vi "DTB_4848_RTU.vi"() -> ()   [LabVIEW 2020]
uses:
  <vilib>/Instr/_visa.llb/VISA Configure Serial Port (Instr).vi
panel:
  in  "Select Device":u16(ring) items=["Broadcast", "DTB4848 1st", "DTB4848 2nd"]
  in  "Boolean 2":bool
  in  "Boolean 3":bool
  in  "Boolean 4":bool
  in  "Boolean 5":bool
  in  "Boolean 6":bool
  in  "Boolean 7":bool
  in  "Boolean 8":bool
  in  "Boolean 9":bool
  in  "Set Point":dbl
  in  "Mode Control":u16
  in  "Ti Integral time":dbl
  in  "Control Cycle 1st":dbl
  in  "Control Cycle 2nd":dbl
  in  "PB Proportional band":dbl
  in  "Td Derivative time":dbl
  in  "Proportional control\noffset error value":dbl
  out "Process Value":dbl
  out "Set Point":dbl
  out "PB Proportional band":dbl
  out "Proportional control\noffset error value":dbl
  out "Control method":u16=13
  out "Ti Integral time":u16=13
  out "Td Derivative time":u16=13
  out "Control Cycle 1st":dbl
  out "Control Cycle 2nd":dbl
  out "Process Value":dbl
  out "Set Point":dbl
  out "PB Proportional band":dbl
  out "Proportional control\noffset error value":dbl
  out "Control method":u16=13
  out "Ti Integral time":u16=13
  out "Td Derivative time":u16=13
  out "Control Cycle 1st":dbl
  out "Control Cycle 2nd":dbl
  out "k":i32
  out "x = 0?":bool
  in  "stop":bool
  in  "Cluster":T1={"VISA resource name"="COM1", "Baud rate"=9600, "Data bits"=8, "Parity"=enum."None", "Stop bits"=10, "Flow control"=0, "Timeout"=1000, "Termination char\n(0xA = '\\n' = LF) "=10, "Enable Termination\nChar (T)"=TRUE} {"Termination char\n(0xA = '\\n' = LF)" format="%.0x"; "Flow control" items=["None", "XON/XOFF", "RTS/CTS", "XON/XOFF & RTS/CTS", "DTR/DSR", "XON/XOFF & DTR/DSR"]; "Stop bits" items=["1.0"=10, "1.5"=15, "2.0"=20]; "Data bits" min=5 max=8 step=1}
  in  "Set":bool
  # "HE THONG DIEU KHIEN GIAM SAT THIET BI DIEU KHIEN NHIET DO DTB4848"
  # "CAU HINH\nTRUYEN THONG"
  # "THIET LAP\nGIA TRI THAM SO"
  # "DTB4848\nDEVICE 1"
  # "DTB4848\nDEVICE 2"
  # "HANH DONG"
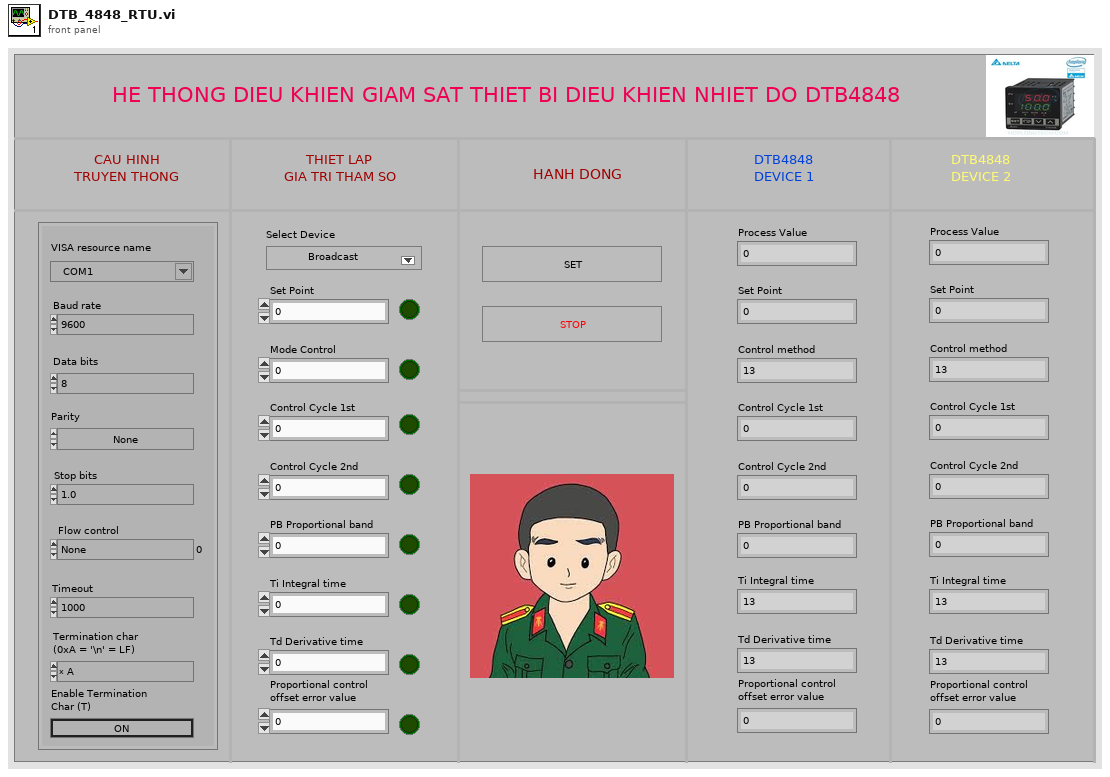
[diagram p1: front panel]
types:
  T1 = cluster{"VISA resource name":refnum<visa-resource-name>, "Baud rate":u32, "Data bits":u16, "Parity":enum16{"None", "Odd", "Even", "Mark", "Space"}, "Stop bits":u16, "Flow control":u16, "Timeout":u32, "Termination char\n(0xA = '\\n' = LF) ":u8, "Enable Termination\nChar (T)":bool}
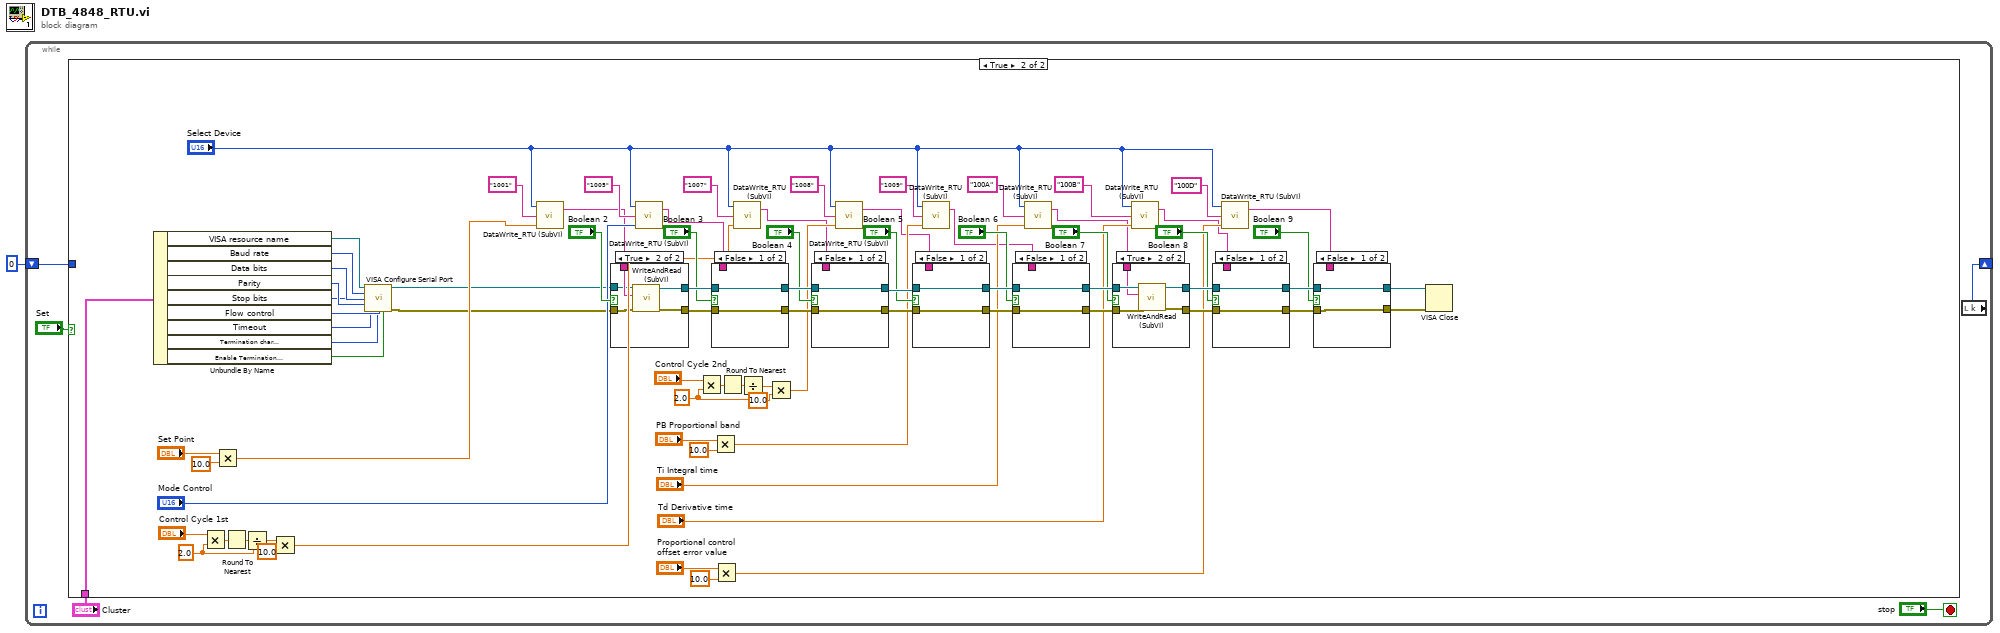
[diagram p0: block diagram]
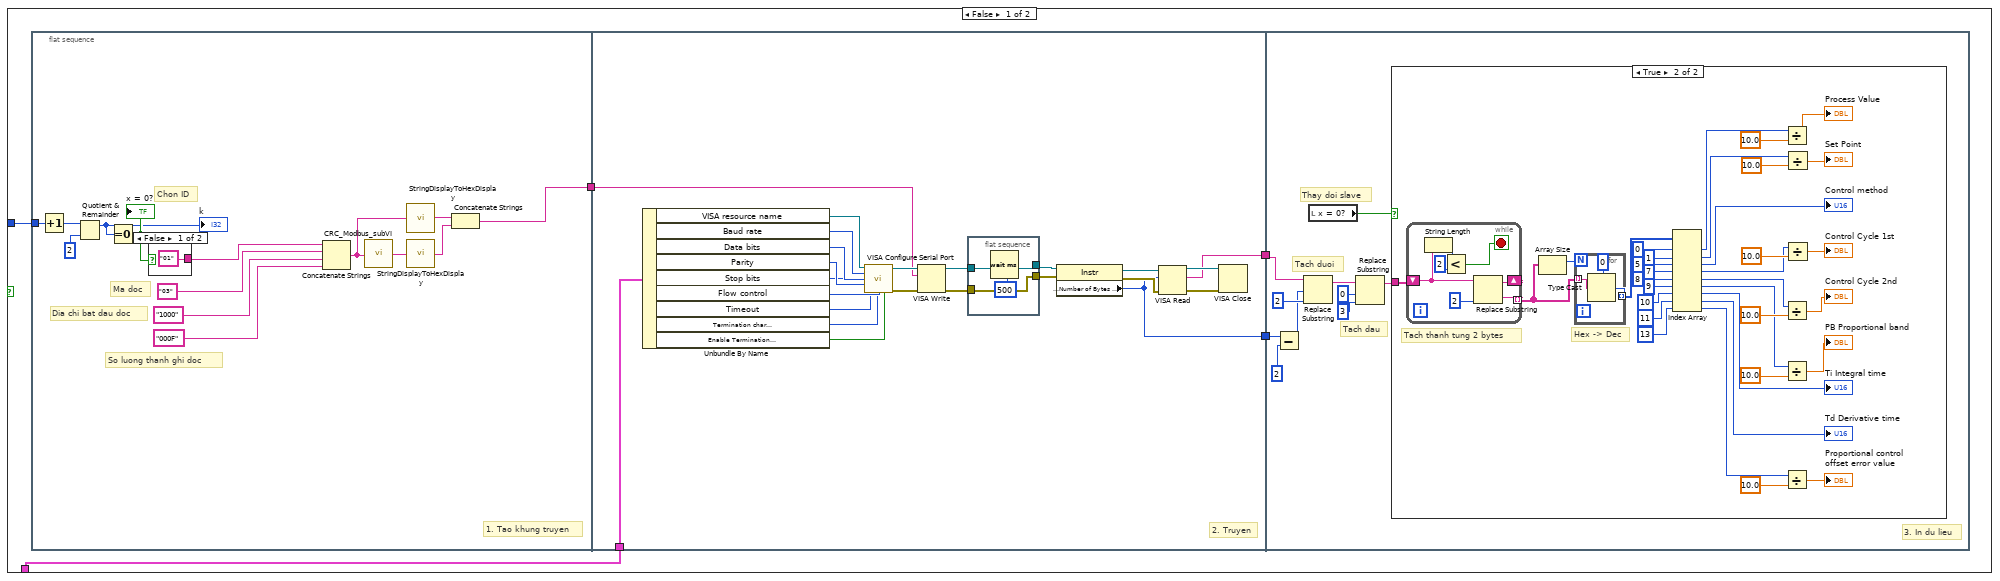
[diagram p2: hidden frame]
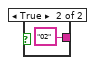
[diagram p3: hidden frame]
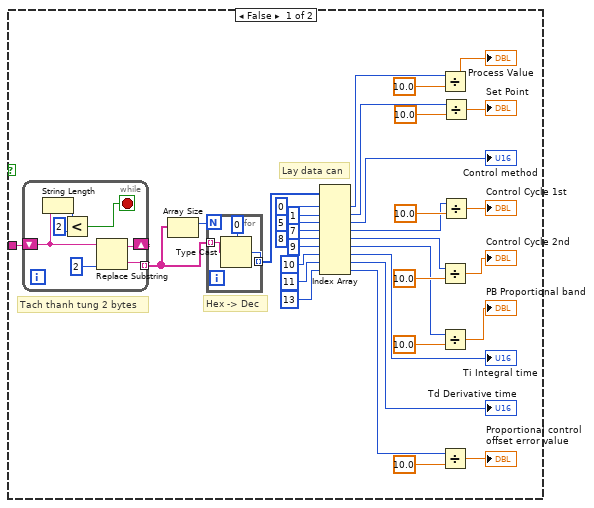
[diagram p4: hidden frame]
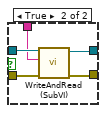
[diagram p5: hidden frame]
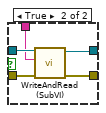
[diagram p6: hidden frame]
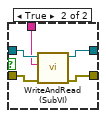
[diagram p8: hidden frame]
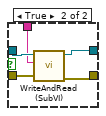
[diagram p9: hidden frame]
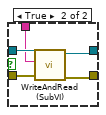
[diagram p10: hidden frame]
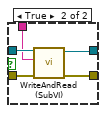
[diagram p11: hidden frame]
diagram:
  n1 = while {
    shift-right: [w5] -> _
    shift-left: 0 ("k") -> [w6]
    stop <- "stop" stop-if-true
    n2 = case shown="True" "Set" {
      tunnel: w6 -> [w11 _]
      tunnel: "Cluster" -> [w10 w230]
      frame False {
        n3 = flat-sequence {
          tunnel: w11 -> [w22]
          tunnel: [w12] -> w7
          tunnel: w10 -> [w31]
          tunnel: [w30] -> w9
          tunnel: [w29] -> w8
          tunnel: w7 -> [w28]
          tunnel: w9 -> [w62]
          tunnel: w8 -> [w56]
          frame #0 {
            # "1. Tao khung truyen"
            # "Chon ID"
            # "So luong thanh ghi doc"
            # "Dia chi bat dau doc"
            # "Ma doc"
            n4 = Increment(x=w22) -> (x+1=w21:i32)
            n5 = Quotient & Remainder(x=w21, y=2) -> (x-y*floor(x/y)=w23:i32)  [unwired: 1 out]
            "k" <- w23
            n6 = Equal To 0?(x=w23) -> (x = 0?=w25:bool)
            "x = 0?" <- w25
            n7 = case shown="False" w25 {
              tunnel: ["01" ("string") "02" ("string")] -> w16
              frame False {
              }
              frame True {
              }
            }
            n8 = Concatenate Strings(w16, "03" ("string"), "1000" ("string"), "000F" ("string")) -> (w17:string)
            n9 = call "CRC_Modbus_subVI.vi"("Before CRC"=w17) -> ("CRC Check"=w20:string)
            n10 = call "StringDisplayToHexDisplay.vi"("Hex Num (Normal Display)"=w17) -> ("Hex Num (Hex Display)"=w19:string)
            n11 = call "StringDisplayToHexDisplay.vi"("Hex Num (Normal Display)"=w20) -> ("Hex Num (Hex Display)"=w18:string)
            n12 = Concatenate Strings(w19, w18) -> (w12:string)
          }
          frame #1 {
            # "2. Truyen"
            n13 = Unbundle By Name(w31) -> ("VISA resource name"=w46:refnum<visa-resource-name>, "Baud rate"=w45:u32, "Data bits"=w44:u16, "Parity"=w43:enum16{"None", "Odd", "Even", "Mark", "Space"}, "Stop bits"=w42:u16, "Flow control"=w41:u16, "Timeout"=w40:u32, "Termination char\n(0xA = '\\n' = LF)"=w39:u8, "Enable Termination\nChar (T)"=w38:bool)
            n14 = call-poly "VISA Configure Serial Port"("VISA resource name"=w46, "timeout (10sec)"=w40, "termination char\n(0xA = '\\n' = LF)"=w39, "Enable Termination\nChar (T)"=w38, "baud rate (9600)"=w45, "data bits (8)"=w44, "parity (0:none)"=w43, "stop bits (10: 1 bit)"=w42, "flow control (0:none)"=w41) -> ("VISA resource name out"=w47:refnum<visa-resource-name>, "error out"=w48:errorcluster)  [unwired: 5 in]
            n15 = VISA Write(VISA resource name=w47, write buffer=w28, error in (no error)=w48) -> (VISA resource name out=w32:refnum<visa-resource-name>, error out=w34:errorcluster)  [unwired: 1 out]
            n16 = flat-sequence {
              tunnel: [w52] -> w35
              tunnel: w34 -> [w52]
              tunnel: [w51] -> w33
              tunnel: w32 -> [w51]
              frame #0 {
                n17 = Wait (ms)(milliseconds to wait=u32 500) -> ()  [unwired: 1 out]
              }
            }
            n18 = property class="Instr"(reference=w33, error in=w35) -> (reference out=w50:refnum<visa-resource-name>, error out=w49:errorcluster, "Serial Settings:Number of Bytes at Serial Port"=w30:u32)
            n19 = VISA Read(VISA resource name=w50, byte count=w30, error in (no error)=w49) -> (VISA resource name out=w37:refnum<visa-resource-name>, read buffer=w29:string, error out=w36:errorcluster)  [unwired: 1 out]
            n20 = VISA Close(VISA resource name=w37, error in (no error)=w36) -> ()  [unwired: 1 out]
          }
          frame #2 {
            # "3. In du lieu"
            # "Thay doi slave"
            # "Tach dau"
            # "Tach duoi"
            n21 = Subtract(x=w62, y=u32 2) -> (x-y=w60:u32)
            n22 = Replace Substring(2:2 ("length (rest)"), 3:w60, 5:w56) -> (1:w54:string)  [unwired: 1 in, 1 out]
            n23 = local read "x = 0?"() -> (w57:bool)
            n24 = Replace Substring(2:3 ("length (rest)"), 3:0 ("offset (0)"), 5:w54) -> (1:w55:string)  [unwired: 1 in, 1 out]
            n25 = case shown="True" w57 {
              tunnel: w55 -> [w64 w109]
              frame False {
                # "Lay data can"
                # "Hex -> Dec"
                # "Tach thanh tung 2 bytes"
                n26 = while {
                  tunnel: [w104] -> w96 mode=indexing
                  shift-right: [w102] -> _
                  shift-left: w64 -> [w101]
                  stop <- w98 stop-if-true
                  n27 = String Length(string=w101) -> (length=w100:i32)
                  n28 = Less?(x=w100, y=2) -> (x < y?=w98:bool)
                  n29 = Replace Substring(2:2 ("length (len. of substring)"), 5:w101) -> (0:w104:string, 1:w102:string)  [unwired: 2 in]
                }
                n30 = Array Size(array=w96) -> (size(s)=w97:i32)
                n31 = for {
                  N: w97 -> [_]
                  tunnel: [w107] -> w95 mode=indexing
                  tunnel: w96 -> [w106] mode=indexing
                  n32 = Type Cast(type=u16 0, x=w106) -> (*(type *) &x=w107:u16)
                }
                n33 = Index Array(array=w95, index #1=0 ("index"), index #2=1 ("index"), index #3=5 ("index"), index #4=7 ("index"), index #5=8 ("index"), index #6=9 ("index"), index #7=10 ("index"), index #8=11 ("index"), index #9=13 ("index")) -> (element #1=w73:u16, element #2=w72:u16, element #3=→"Control method":u16, element #4=w70:u16, element #5=w69:u16, element #6=w68:u16, element #7=→"Ti Integral time":u16, element #8=→"Td Derivative time":u16, element #9=w65:u16)
                n34 = Divide(x=w73, y=10.0) -> (x/y=→"Process Value":dbl)
                n35 = Divide(x=w69, y=10.0) -> (x/y=→"Control Cycle 2nd":dbl)
                n36 = Divide(x=w68, y=10.0) -> (x/y=→"PB Proportional band":dbl)
                n37 = Divide(x=w65, y=10.0) -> (x/y=→"Proportional control\noffset error value":dbl)
                n38 = Divide(x=w72, y=10.0) -> (x/y=→"Set Point":dbl)
                n39 = Divide(x=w70, y=10.0) -> (x/y=→"Control Cycle 1st":dbl)
              }
              frame True {
                # "Hex -> Dec"
                # "Tach thanh tung 2 bytes"
                n40 = while {
                  tunnel: [w148] -> w110 mode=indexing
                  shift-right: [w146] -> _
                  shift-left: w109 -> [w145]
                  stop <- w142 stop-if-true
                  n41 = String Length(string=w145) -> (length=w144:i32)
                  n42 = Less?(x=w144, y=2) -> (x < y?=w142:bool)
                  n43 = Replace Substring(2:2 ("length (len. of substring)"), 5:w145) -> (0:w148:string, 1:w146:string)  [unwired: 2 in]
                }
                n44 = Array Size(array=w110) -> (size(s)=w111:i32)
                n45 = for {
                  N: w111 -> [_]
                  tunnel: [w151] -> w108 mode=indexing
                  tunnel: w110 -> [w150] mode=indexing
                  n46 = Type Cast(type=u16 0, x=w150) -> (*(type *) &x=w151:u16)
                }
                n47 = Index Array(array=w108, index #1=0 ("index"), index #2=1 ("index"), index #3=5 ("index"), index #4=7 ("index"), index #5=8 ("index"), index #6=9 ("index"), index #7=10 ("index"), index #8=11 ("index"), index #9=13 ("index")) -> (element #1=w120:u16, element #2=w119:u16, element #3=→"Control method":u16, element #4=w117:u16, element #5=w116:u16, element #6=w115:u16, element #7=→"Ti Integral time":u16, element #8=→"Td Derivative time":u16, element #9=w112:u16)
                n48 = Divide(x=w120, y=10.0) -> (x/y=→"Process Value":dbl)
                n49 = Divide(x=w116, y=10.0) -> (x/y=→"Control Cycle 2nd":dbl)
                n50 = Divide(x=w115, y=10.0) -> (x/y=→"PB Proportional band":dbl)
                n51 = Divide(x=w112, y=10.0) -> (x/y=→"Proportional control\noffset error value":dbl)
                n52 = Divide(x=w119, y=10.0) -> (x/y=→"Set Point":dbl)
                n53 = Divide(x=w117, y=10.0) -> (x/y=→"Control Cycle 1st":dbl)
              }
            }
          }
        }
      }
      frame True {
        w184 = 2.0 ("y")
        w194 = 2.0 ("y")
        n54 = Unbundle By Name(w230) -> ("VISA resource name"=w229:refnum<visa-resource-name>, "Baud rate"=w228:u32, "Data bits"=w227:u16, "Parity"=w226:enum16{"None", "Odd", "Even", "Mark", "Space"}, "Stop bits"=w225:u16, "Flow control"=w224:u16, "Timeout"=w223:u32, "Termination char\n(0xA = '\\n' = LF)"=w222:u8, "Enable Termination\nChar (T)"=w221:bool)
        n55 = Multiply(x="Control Cycle 1st", y=w194) -> (x*y=w191:dbl)
        n56 = Multiply(x="Set Point", y=10.0) -> (x*y=w169:dbl)
        n57 = Round To Nearest(number=w191) -> (nearest integer value=w193:dbl)
        n58 = Divide(x=w193, y=w194) -> (x/y=w192:dbl)
        n59 = Multiply(x=w192, y=10.0) -> (x*y=w167:dbl)
        n60 = call-poly "VISA Configure Serial Port"("VISA resource name"=w229, "timeout (10sec)"=w223, "termination char\n(0xA = '\\n' = LF)"=w222, "Enable Termination\nChar (T)"=w221, "baud rate (9600)"=w228, "data bits (8)"=w227, "parity (0:none)"=w226, "stop bits (10: 1 bit)"=w225, "flow control (0:none)"=w224) -> ("VISA resource name out"=w153:refnum<visa-resource-name>, "error out"=w152:errorcluster)  [unwired: 5 in]
        n61 = call "DataWrite_RTU (SubVI).vi"("Data"=w169, "Address"="1001", "Select Device"="Select Device") -> ("Write frame"=w161:string)  [unwired: 1 out]
        n62 = case shown="True" "Boolean 2" {
          tunnel: [w281 w286] -> w213
          tunnel: [w280 w285] -> w205
          tunnel: w161 -> [_ w284]
          tunnel: w153 -> [w281 w283]
          tunnel: w152 -> [w280 w282]
          frame False {
          }
          frame True {
            n63 = call "WriteAndRead (SubVI).vi"("error in (no error)"=w282, "Write"=w284, "VISA Refnum in"=w283) -> ("error out"=w285:errorcluster, "VISA resource name out"=w286:refnum<visa-resource-name>)  [unwired: 7 in]
          }
        }
        n64 = call "DataWrite_RTU (SubVI).vi"("Data"="Mode Control", "Address"="1005", "Select Device"="Select Device") -> ("Write frame"=w160:string)  [unwired: 1 out]
        n65 = Multiply(x="Control Cycle 2nd", y=w184) -> (x*y=w188:dbl)
        n66 = case shown="False" "Boolean 3" {
          tunnel: [w274 w277] -> w214
          tunnel: w213 -> [w274 w278]
          tunnel: [w273 w276] -> w206
          tunnel: w205 -> [w273 w279]
          tunnel: w160 -> [_ w275]
          frame False {
          }
          frame True {
            n67 = call "WriteAndRead (SubVI).vi"("error in (no error)"=w279, "Write"=w275, "VISA Refnum in"=w278) -> ("error out"=w276:errorcluster, "VISA resource name out"=w277:refnum<visa-resource-name>)  [unwired: 7 in]
          }
        }
        n68 = Multiply(x="PB Proportional band", y=10.0) -> (x*y=w165:dbl)
        n69 = Multiply(x="Proportional control\noffset error value", y=10.0) -> (x*y=w162:dbl)
        n70 = Round To Nearest(number=w188) -> (nearest integer value=w186:dbl)
        n71 = call "DataWrite_RTU (SubVI).vi"("Data"=w167, "Address"="1007", "Select Device"="Select Device") -> ("Write frame"=w159:string)  [unwired: 1 out]
        n72 = Divide(x=w186, y=w184) -> (x/y=w187:dbl)
        n73 = Multiply(x=w187, y=10.0) -> (x*y=w166:dbl)
        n74 = case shown="False" "Boolean 4" {
          tunnel: [w267 w271] -> w215
          tunnel: w214 -> [w267 w272]
          tunnel: [w266 w269] -> w207
          tunnel: w206 -> [w266 w270]
          tunnel: w159 -> [_ w268]
          frame False {
          }
          frame True {
            n75 = call "WriteAndRead (SubVI).vi"("error in (no error)"=w270, "Write"=w268, "VISA Refnum in"=w272) -> ("error out"=w269:errorcluster, "VISA resource name out"=w271:refnum<visa-resource-name>)  [unwired: 7 in]
          }
        }
        n76 = call "DataWrite_RTU (SubVI).vi"("Data"=w166, "Address"="1008", "Select Device"="Select Device") -> ("Write frame"=w158:string)  [unwired: 1 out]
        n77 = case shown="False" "Boolean 5" {
          tunnel: [w260 w264] -> w216
          tunnel: w215 -> [w260 w265]
          tunnel: [w259 w262] -> w208
          tunnel: w207 -> [w259 w263]
          tunnel: w158 -> [_ w261]
          frame False {
          }
          frame True {
            n78 = call "WriteAndRead (SubVI).vi"("error in (no error)"=w263, "Write"=w261, "VISA Refnum in"=w265) -> ("error out"=w262:errorcluster, "VISA resource name out"=w264:refnum<visa-resource-name>)  [unwired: 7 in]
          }
        }
        n79 = call "DataWrite_RTU (SubVI).vi"("Data"=w165, "Address"="1009", "Select Device"="Select Device") -> ("Write frame"=w157:string)  [unwired: 1 out]
        n80 = case shown="False" "Boolean 6" {
          tunnel: [w253 w257] -> w217
          tunnel: w216 -> [w253 w258]
          tunnel: [w252 w255] -> w209
          tunnel: w208 -> [w252 w256]
          tunnel: w157 -> [_ w254]
          frame False {
          }
          frame True {
            n81 = call "WriteAndRead (SubVI).vi"("error in (no error)"=w256, "Write"=w254, "VISA Refnum in"=w258) -> ("error out"=w255:errorcluster, "VISA resource name out"=w257:refnum<visa-resource-name>)  [unwired: 7 in]
          }
        }
        n82 = call "DataWrite_RTU (SubVI).vi"("Data"="Ti Integral time", "Address"="100A", "Select Device"="Select Device") -> ("Write frame"=w156:string)  [unwired: 1 out]
        n83 = case shown="True" "Boolean 7" {
          tunnel: [w246 w251] -> w218
          tunnel: w217 -> [w246 w250]
          tunnel: [w245 w248] -> w210
          tunnel: w209 -> [w245 w249]
          tunnel: w156 -> [_ w247]
          frame False {
          }
          frame True {
            n84 = call "WriteAndRead (SubVI).vi"("error in (no error)"=w249, "Write"=w247, "VISA Refnum in"=w250) -> ("error out"=w248:errorcluster, "VISA resource name out"=w251:refnum<visa-resource-name>)  [unwired: 7 in]
          }
        }
        n85 = call "DataWrite_RTU (SubVI).vi"("Data"="Td Derivative time", "Address"="100B", "Select Device"="Select Device") -> ("Write frame"=w155:string)  [unwired: 1 out]
        n86 = case shown="False" "Boolean 8" {
          tunnel: [w239 w243] -> w219
          tunnel: w218 -> [w239 w244]
          tunnel: [w238 w241] -> w211
          tunnel: w210 -> [w238 w242]
          tunnel: w155 -> [_ w240]
          frame False {
          }
          frame True {
            n87 = call "WriteAndRead (SubVI).vi"("error in (no error)"=w242, "Write"=w240, "VISA Refnum in"=w244) -> ("error out"=w241:errorcluster, "VISA resource name out"=w243:refnum<visa-resource-name>)  [unwired: 7 in]
          }
        }
        n88 = call "DataWrite_RTU (SubVI).vi"("Data"=w162, "Address"="100D", "Select Device"="Select Device") -> ("Write frame"=w154:string)  [unwired: 1 out]
        n89 = case shown="False" "Boolean 9" {
          tunnel: [w232 w236] -> w220
          tunnel: w219 -> [w232 w237]
          tunnel: [w231 w234] -> w212
          tunnel: w211 -> [w231 w235]
          tunnel: w154 -> [_ w233]
          frame False {
          }
          frame True {
            n90 = call "WriteAndRead (SubVI).vi"("error in (no error)"=w235, "Write"=w233, "VISA Refnum in"=w237) -> ("error out"=w234:errorcluster, "VISA resource name out"=w236:refnum<visa-resource-name>)  [unwired: 7 in]
          }
        }
        n91 = VISA Close(VISA resource name=w220, error in (no error)=w212) -> ()  [unwired: 1 out]
      }
    }
    n92 = local read "k"() -> (w5:i32)
  }
